vi "Report Gen Item.vi"(8 "error in (no error)":errorcluster, 10 "Error Info":T1 {"Context"."name" items=["Method Name", "Parameter Name", "VI Name", "Control Name", "Proxy Dll Path", "Project Library Name"]; "Error Number" items=["ERR_NOERROR"=0, "ERR_ACCESS_OUTPUTFOLDER"=1, "ERR_INVALID_LIBRARYNAME"=2, "ERR_CREATE_VIWRAPPER"=3, "ERR_UNKNOWN"=201, "ERR_BAD_ARGUMENT"=202, "ERR_URL_NOTFOUND_BADWSDL"=203, "ERR_BADLYFORMATTEDURL"=204, "ERR_BADHOSTNAME"=205, "ERR_BADDIRECTORY"=206, "ERR_UNAUTHORIZEDACCESS"=207, "ERR_CREATELIBRARY"=208, "ERR_COMPILEERROR"=209]}, 11 "report":T5) -> (0 "error out":errorcluster, 3 "report out":T5)   [LabVIEW 2020, in "WebServiceImporter.lvlib" / "Error Handling.lvlib"]
uses:
  <vilib>/Platform/WebService/Error Handling/Error Handling.lvlib
  <resource>/importtools/NISH Report/Generate Report Object Reference.ctl
  <vilib>/Platform/WebService/Error Handling/Error/Error Info.ctl
  <vilib>/Platform/WebService/Error Handling/Error/Error Number.ctl
  <vilib>/Platform/WebService/Error Handling/Error/Context.ctl
  <vilib>/Platform/WebService/Error Handling/Error/Context Name.ctl
  <resource>/importtools/NISH Report/NISH Report.lvlib
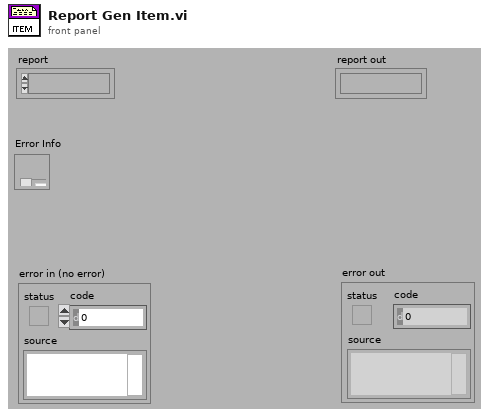
[diagram p1: front panel]
types:
  T1 = typedef "WebServiceImporter.lvlib/Error Handling.lvlib/Error Info.ctl" = cluster{"Specifics":string, "Error Number":T2, "Call Chain":string, "Context":T3}
  T2 = typedef "WebServiceImporter.lvlib/Error Handling.lvlib/Error Number.ctl" = u16
  T3 = typedef "WebServiceImporter.lvlib/Error Handling.lvlib/Context.ctl" = cluster{"name":T4, "value":string}[]
  T4 = typedef "WebServiceImporter.lvlib/Error Handling.lvlib/Context Name.ctl" = u16
  T5 = typedef "NISH Report.lvlib/Generate Report Object Reference.ctl" = refnum<k1>
  T6 = cluster{"Italic":enum16{"Italic Unchanged", "Italic On", "Italic Off"}, "Strike Through":enum16{"Strike Through Unchanged", "Strike Through On", "Strike Through Off"}, "Underline":enum16{"Underline Unchanged", "Underline On", "Underline Off"}, "Bold":enum16{"Bold Unchanged", "Bold On", "Bold Off"}}
  T7 = cluster{"Charset (-1)":i16, "Weight (-1)":i16, "Name":string, "Size":string}
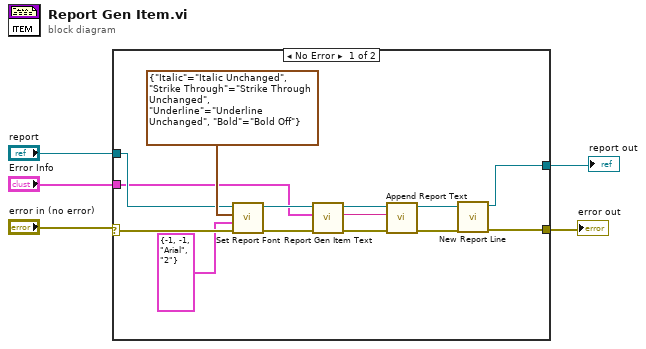
[diagram p0: block diagram]
diagram:
  n1 = case shown="No Error" "error in (no error)" {
    selector: "error in (no error)" -> [w19 w20]
    tunnel: "Error Info" -> [w14 _]
    tunnel: "report" -> [w16 w21]
    tunnel: [w7 w20] -> w2
    tunnel: [w6 w21] -> w1
    frame No Error {
      n2 = call <resource>:"Set Report Font.vi"("error in (no error)"=w19, "font settings"=T7 {"Charset (-1)"=-1, "Weight (-1)"=-1, "Name"="Arial", "Size"="2"} ("Font Settings"), "text options"=T6 {"Italic"=enum."Italic Unchanged", "Strike Through"=enum."Strike Through Unchanged", "Underline"=enum."Underline Unchanged", "Bold"=enum."Bold Off"} ("Text Options"), "report in"=w16) -> ("error out"=w13:errorcluster, "report out"=w15:T5)  [unwired: 3 in]
      n3 = call <vilib>:"Report Gen Item Text.vi"("error in (no error)"=w13, "Error Info"=w14, "report"=w15) -> ("error out"=w10:errorcluster, "Text out"=w11:string, "report out"=w12:T5)  [unwired: 6 in]
      n4 = call <resource>:"Append Report Text.vi"("error in (no error)"=w10, "text"=w11, "report in"=w12) -> ("error out"=w8:errorcluster, "report out"=w9:T5)  [unwired: 3 in]
      n5 = call <resource>:"New Report Line.vi"("error in (no error)"=w8, "report in"=w9) -> ("error out"=w7:errorcluster, "report out"=w6:T5)  [unwired: 4 in]
    }
    frame Error {
    }
  }
  "report out" <- w1
  "error out" <- w2
